vi "Simulation Configuration Write.vi"(8 "error in (no error)":errorcluster, 10 "configuration":path=path "simulation configuration.ini", 11 "simulation configuration":T1={"maxTime"=5.0, "enableVisualization"=TRUE, "statechart"=path "iRobot Navigation State Machine.vi", "environment"=path "iRobot Navigation State Machine.vi", "record"=path "Simulation Record.xml", "autograde?"=TRUE, "interactive?"=FALSE, "feedback mode"=enum."debug navigation"}) -> (0 "error out":errorcluster)   [LabVIEW 2013]
uses:
  CyberSim interface/Simulation Configuration.ctl
  autograder/feedbackMode.ctl
  <vilib>/Utility/config.llb/Write Key (Path).vi
  <vilib>/Utility/config.llb/Write Key (I32).vi
  <vilib>/Utility/config.llb/NI_LVConfig.lvlib
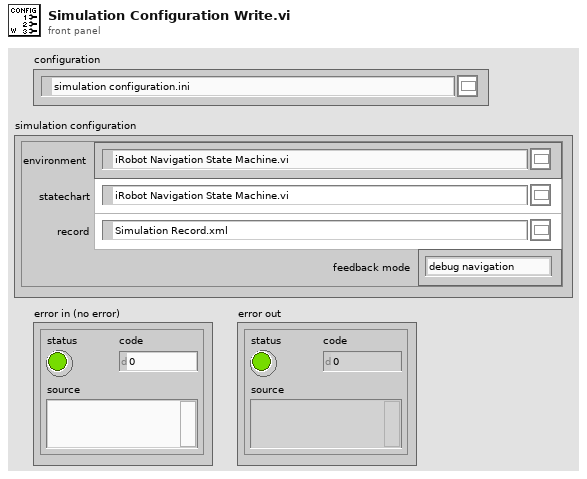
[diagram p1: front panel]
types:
  T1 = typedef "Simulation Configuration.ctl" = cluster{"maxTime":sgl, "enableVisualization":bool, "statechart":path, "environment":path, "record":path, "autograde?":bool, "interactive?":bool, "feedback mode":T2}
  T2 = typedef "feedbackMode.ctl" = enum32{"debug navigation", "debug hill climb", "autograde navigation", "autograde hill climb"}
  T3 = typedef "NI_LVConfig.lvlib/Config Data RefNum.ctl" = refnum<k1>
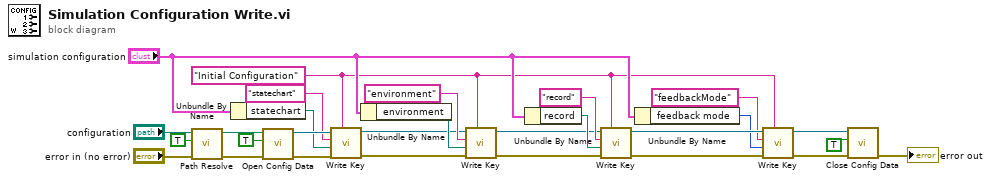
[diagram p0: block diagram]
diagram:
  w5 = "Initial Configuration" ("section")
  n1 = call "Path Resolve.vi"("Error In"="error in (no error)", "create?"=TRUE, "absolute or relative path"="configuration") -> ("Error Out"=w17:errorcluster, "resolved path"=w18:path)  [unwired: 7 in]
  n2 = Unbundle By Name("simulation configuration") -> ("statechart"=w24:path)
  n3 = call <vilib>:"Open Config Data.vi"("error in (no error)"=w17, "create file if necessary (T)"=TRUE, "configuration file path"=w18) -> ("error out"=w27:errorcluster, "refnum"=w26:T3)  [unwired: 6 in, 1 out]
  n4 = call-poly <vilib>:"Write Key.vi"("section"=w5, "error in (no error)"=w27, "value"=w24, "key"="statechart", "refnum"=w26) -> ("error out"=w13:errorcluster, "refnum out"=w14:T3)  [unwired: 4 in, 1 out]
  n5 = Unbundle By Name("simulation configuration") -> ("environment"=w22:path)
  n6 = call-poly <vilib>:"Write Key.vi"("section"=w5, "error in (no error)"=w13, "value"=w22, "key"="environment", "refnum"=w14) -> ("error out"=w1:errorcluster, "refnum out"=w2:T3)  [unwired: 4 in, 1 out]
  n7 = Unbundle By Name("simulation configuration") -> ("record"=w11:path)
  n8 = call-poly <vilib>:"Write Key.vi"("section"=w5, "error in (no error)"=w1, "value"=w11, "key"="record", "refnum"=w2) -> ("error out"=w9:errorcluster, "refnum out"=w10:T3)  [unwired: 4 in, 1 out]
  n9 = Unbundle By Name("simulation configuration") -> ("feedback mode"=w7:T2)
  n10 = call-poly <vilib>:"Write Key.vi"("section"=w5, "error in (no error)"=w9, "value"=w7, "key"="feedbackMode", "refnum"=w10) -> ("error out"=w3:errorcluster, "refnum out"=w4:T3)  [unwired: 4 in, 1 out]
  n11 = call <vilib>:"Close Config Data.vi"("error in (no error)"=w3, "write file if changed (T)"=TRUE, "refnum"=w4) -> ("error out"=→"error out":errorcluster)  [unwired: 7 in, 1 out]
